vi "Connect.vi"(8 "error in (no error)":errorcluster, 9 "timeout_ms (-1)":i32=-1, 11 "INetworkReader in":refnum<class "INetworkReader.lvclass">) -> (0 "error out":errorcluster, 3 "INetworkReader out":refnum<class "INetworkReader.lvclass">)   [LabVIEW 2024, in "INetworkReader.lvclass"]
uses:
  INetworkReader.lvclass
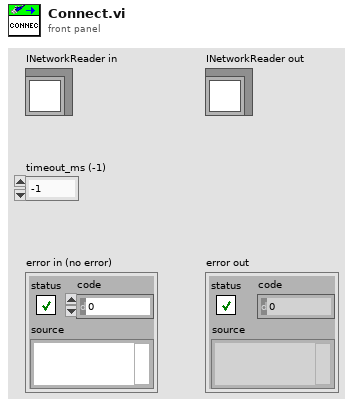
[diagram p1: front panel]
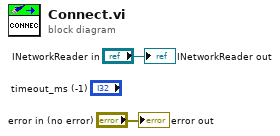
[diagram p0: block diagram]
diagram:
  "error out" <- "error in (no error)"
  "INetworkReader out" <- "INetworkReader in"
